vi "Fire ProcessingStateChanged Event_DAQ.vi"(8 "error in (no error)":errorcluster, 10 "DAQState":variant, 11 "Main in":refnum<class "Main.lvclass">) -> (0 "error out":errorcluster, 3 "Main out":refnum<class "Main.lvclass">)   [LabVIEW 2019, in "Main.lvclass"]
doc: "Developed by Kevin Thompson\nkevin@thompsonengineering.net\n\nCopyright 2018-2020\nThompson Engineering, LLC"
uses:
  Main.lvclass
  DataTypes/ProcessingState--enum.ctl
  DataTypes/ProcessingStateChg EvData--cluster.ctl
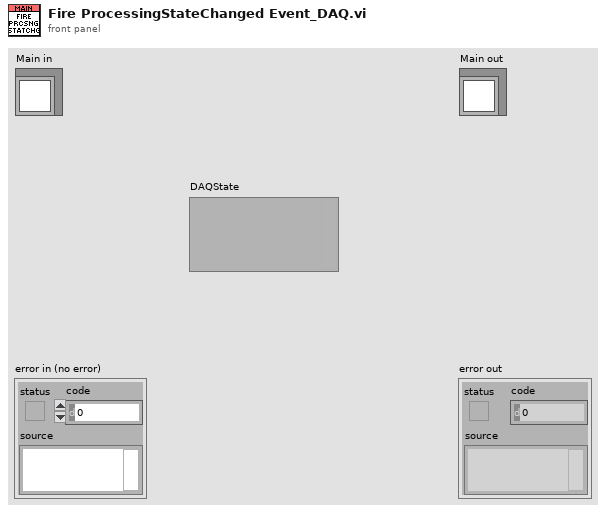
[diagram p1: front panel]
types:
  T1 = typedef "Main.lvclass/ProcessingStateChg EvData--cluster.ctl" = cluster{"Time Stamp":timestamp, "OLD ProcessingState":T2, "NEW ProcessingState":T2}
  T2 = typedef "Main.lvclass/ProcessingState--enum.ctl" = enum16{"Idle", "Starting", "Running", "Done", "Error"}
  T3 = typedef "Main.lvclass/Public Events--cluster.ctl" = cluster{"Main.AsyncCmd Event":refnum<user-event>, "Main.AsyncMsg Event":refnum<user-event>, "stop process":refnum<user-event>, "UpdateControlValue Ev":refnum<user-event>, "ProcessingStateChg Ev":refnum<user-event>}
  T4 = typedef "ProcessingState--enum.ctl" = enum16{"Idle", "Starting", "Running", "Done", "Error"}
  T5 = typedef "Type Descriptor Enumeration__ogtk.ctl" = enum8{"<Null>", "I8", "I16", "I32", "I64", "U8", "U16", "U32", "U64", "SGL", "DBL", "EXT", "CSG", "CDB", "CXT", "0x0F", "0x10", "0x11", "0x12", "0x13", "0x14", "Enum U8", "Enum U16", "Enum U32", "Enum U64", "SGL PQ", "DBL PQ", "EXT PQ", "CSG PQ", "CDB PQ", "CXT PQ", "0x1F", "0x20", "Boolean", "0x22", "0x23", "0x24", "0x25", "0x26", "0x27", "0x28", "0x29", "0x2A", "0x2B", "0x2C", "0x2D", "0x2E", "0x2F", "String", "0x31", "Path", "Pict", "0x34", "0x35", "0x36", "DAQ", "0x38", "0x39", "0x3A", "0x3B", "0x3C", "0x3D", "0x3E", "0x3F", "Array", "0x41", "0x42", "0x43", "0x44", "0x45", "0x46", "0x47", "0x48", "0x49", "0x4A", "0x4B", "0x4C", "0x4D", "0x4E", "0x4F", "Cluster", "0x51", "0x52", "Variant", "Waveform", "0x55", "0x56", "0x57", "0x58", "0x59", "0x5A", "0x5B", "0x5C", "0x5D", "0x5E", "0x5F", "0x60", "0x61", "0x62", "0x63", "0x64", "0x65", "0x66", "0x67", "0x68", "0x69", "0x6A", "0x6B", "0x6C", "0x6D", "0x6E", "0x6F", "Refnum"}
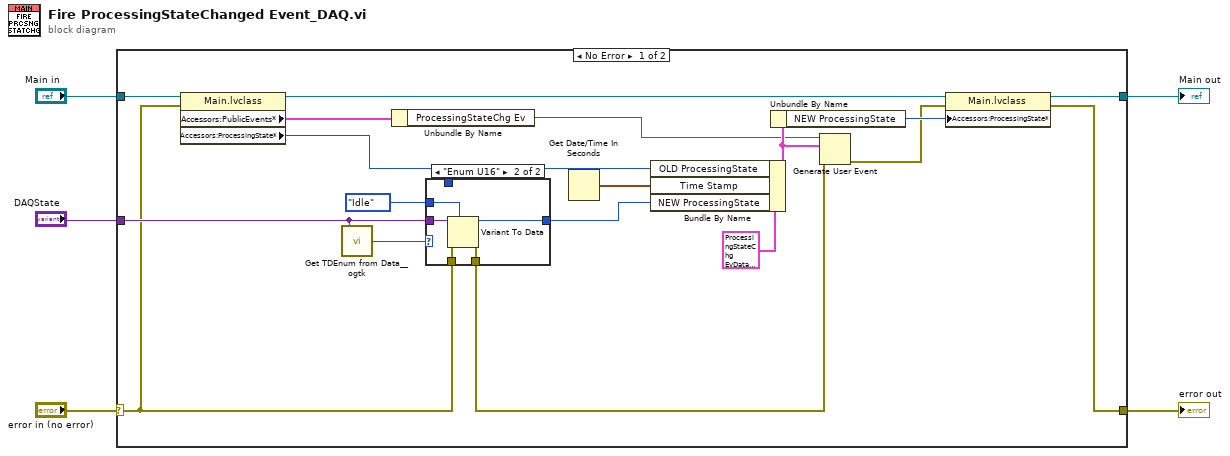
[diagram p0: block diagram]
diagram:
  n1 = case shown="No Error" "error in (no error)" {
    selector: "error in (no error)" -> [w12 w32]
    tunnel: [w13 w32] -> w4
    tunnel: [w17 w31] -> w2
    tunnel: "Main in" -> [w22 w31]
    tunnel: "DAQState" -> [w20 _]
    frame No Error {
      n2 = property class="Main.lvclass"(reference=w22, error in=w12) -> (reference out=w9:refnum<class "Main.lvclass">, "Accessors:PublicEvents*"=w10:T3, "Accessors:ProcessingState*"=w8:T4)  [unwired: 1 out]
      n3 = call <userlib>:"Get TDEnum from Data__ogtk.vi"("Data"=w20) -> ("Type Descriptor Enumeration"=w21:T5)  [unwired: 4 in]
      n4 = Unbundle By Name(w10) -> ("ProcessingStateChg Ev"=w11:refnum<user-event>)
      n5 = case shown="\"Enum U16\"" w21 {
        tunnel: w8 -> [w24 _]
        tunnel: w20 -> [_ w30]
        tunnel: [w24 w29] -> w19
        tunnel: ProcessingState--enum."Idle" ("ProcessingState") -> [_ w28]
        tunnel: w12 -> [w25 w27]
        tunnel: [w25 w26] -> w18
        frame "<Null>", Default {
        }
        frame "Enum U16" {
          n6 = Variant To Data(error in=w27, type=w28, Variant=w30) -> (data=w29:T2, error out=w26:errorcluster)
        }
      }
      n7 = Get Date/Time In Seconds() -> (seconds since 1Jan1904=w23:timestamp)
      n8 = Bundle By Name(cluster=T1 {"Time Stamp"=timestamp(0 s since 1904-01-01), "OLD ProcessingState"=enum."Idle", "NEW ProcessingState"=enum."Idle"} ("DAQAcqModeChg EvData"), "OLD ProcessingState"=w8, "Time Stamp"=w23, "NEW ProcessingState"=w19) -> (w16:T1)
      n9 = Unbundle By Name(w16) -> ("NEW ProcessingState"=w15:T2)
      n10 = Generate User Event(user event=w11, event data cluster=w16, error in=w18) -> (error out=w14:errorcluster)  [unwired: 1 in, 1 out]
      n11 = property class="Main.lvclass"(reference=w9, error in=w14, "Accessors:ProcessingState*"=w15) -> (reference out=w17:refnum<class "Main.lvclass">, error out=w13:errorcluster)
    }
    frame Error {
    }
  }
  "error out" <- w4
  "Main out" <- w2
